vi "DigitalOutCommand.vi"(0 "error in":errorcluster, 2 "Parameters":cluster{"Component name":u16, "State":bool} {"Component name" items=["left_itb_light_inner", "right_itb_light_inner", "torso_left_itb_light_inner", "torso_right_itb_light_inner", "left_itb_light_outer", "right_itb_light_outer", "torso_left_itb_light_outer", "torso_right_itb_light_outer"]}, 3 "node":string) -> (1 "error out":errorcluster)   [LabVIEW 2012]
doc: "Write digital output to Baxters"
uses:
  <userlib>/ROS for LabVIEW Software/ROS/Code/Console/Servers/ServerSubs/TopicDef.ctl
  <userlib>/ROS for LabVIEW Software/ROS/Code/SubVIs/_ROSDirection.ctl
panel:
  # "Controls navigator button panels on Baxter's arms and torso"
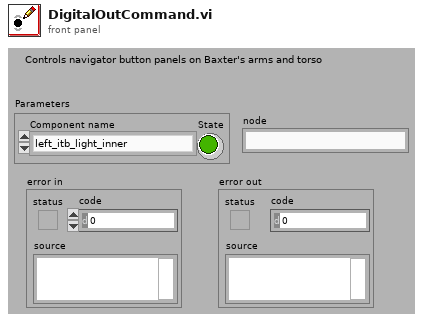
[diagram p1: front panel]
types:
  T1 = typedef "TopicDef.ctl" = cluster{"Topic":string, "Type":string, "Action":T2, "Update (ms)":u16, "queue size":u16}
  T2 = typedef "_ROSDirection.ctl" = enum16{"Node", "Publisher", "Subscriber", "ServiceClient", "ServiceProvider"}
  T3 = typedef "_ROSControl.ctl" = cluster{"topic port":u16, "Node":string, "topic":string, "type":string, "node port":u16, "error ":errorcluster, "Direction":T2, "Update (ms)":u16, "FIFO size":u16}
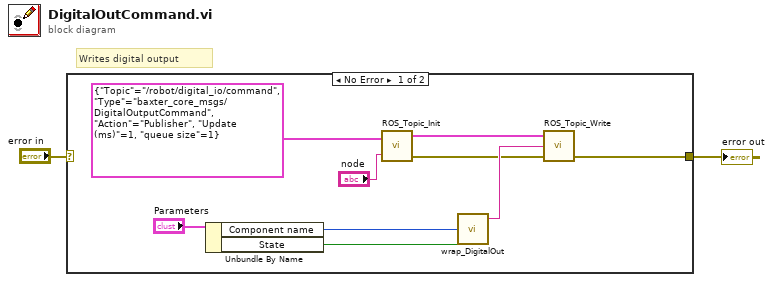
[diagram p0: block diagram]
diagram:
  # "Writes digital output"
  n1 = case shown="No Error" "error in" {
    selector: "error in" -> [_ w12]
    tunnel: [w7 w12] -> w2
    frame No Error {
      n2 = Unbundle By Name("Parameters") -> ("Component name"=w4:u16, "State"=w3:bool)
      n3 = call <userlib>:"ROS_Topic_Init.vi"("Definitions"=T1 {"Topic"="/robot/digital_io/command", "Type"="baxter_core_msgs/DigitalOutputCommand", "Action"=enum."Publisher", "Update (ms)"=1, "queue size"=1}, "node"="node") -> ("ROS out"=w11:T3, "error out"=w6:errorcluster)  [unwired: 1 in]
      n4 = call <userlib>:"wrap_DigitalOut.vi"("State"=w3, "Component ID"=w4) -> ("msg out"=w8:string)  [unwired: 3 in]
      n5 = call <userlib>:"ROS_Topic_Write.vi"("error in (no error)"=w6, "Msg in"=w8, "ROS in"=w11) -> ("error out"=w7:errorcluster)  [unwired: 1 in, 1 out]
    }
    frame Error {
    }
  }
  "error out" <- w2
